vi "2022-LinearInterpolate.vi"(10 "Points":cluster{"X":dbl, "Y":dbl}[](array[cluster]), 11 "Value":dbl) -> (3 "Output":dbl)   [LabVIEW 2019]
doc: "Linearly interpolates between the two points set in config. The sign of the input does not matter."
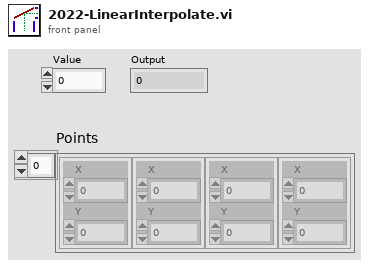
[diagram p1: front panel]
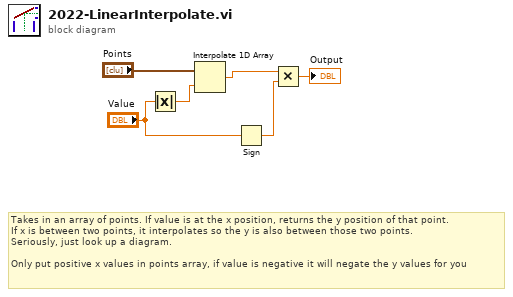
[diagram p0: block diagram]
diagram:
  # "Takes in an array of points. If value is at the x position, returns the y position of that point.\nIf x is between two points, it interpolates so the y is also between those two points.\nSeriously, just look up a diagram.\n\nOnly put positive x values in points array, if value is negative it will negate the y values for you"
  n1 = Absolute Value(x="Value") -> (abs(x)=w4:dbl)
  n2 = Interpolate 1D Array(1:w4, 2:"Points") -> (0:w2:dbl)
  n3 = Sign(1:"Value") -> (0:w6:dbl)
  n4 = Multiply(x=w2, y=w6) -> (x*y=→"Output":dbl)
